vi "getInternalShutdown.vi"(11 "UserEvents in":refnum<class "UserEvents.lvclass">) -> (2 "InternalShutdown":refnum<user-event>, 3 "UserEvents out":refnum<class "UserEvents.lvclass">)   [LabVIEW 2016, in "UserEvents.lvclass"]
uses:
  UserEvents.lvclass
  DataTypes/General/ShutdownEvent.ctl
  UserEvents.lvclass/UserEvents.ctl
  DataTypes/General/M1M3SupportGeneral.lvlib
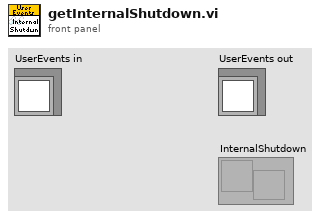
[diagram p1: front panel]
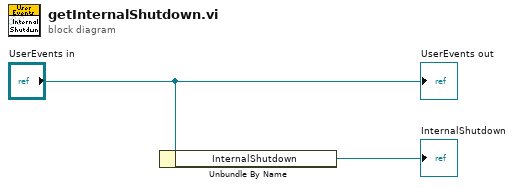
[diagram p0: block diagram]
diagram:
  n1 = Unbundle By Name("UserEvents in") -> ("InternalShutdown"=→"InternalShutdown":refnum<user-event>)
  "UserEvents out" <- "UserEvents in"
